vi "Set A4 Size.vi"(8 "error in (no error)":errorcluster, 10 "File refnum":refnum<k7>) -> (0 "error out":errorcluster, 2 "File refnum out":refnum<k7>)   [LabVIEW 2020, in "lvpptx.lvlib"]
uses:
  lvpptx.lvlib
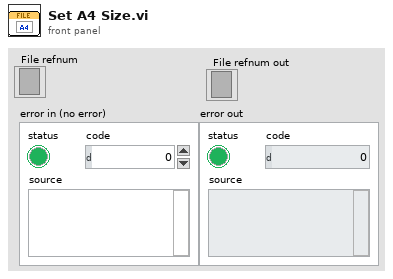
[diagram p1: front panel]
types:
  T1 = cluster{"SlideWidth (inches)":sgl, "SlideHeight (inches)":sgl}
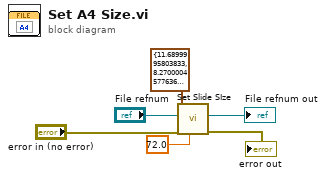
[diagram p0: block diagram]
diagram:
  n1 = call "Set Slide SIze.vi"("DPI"=72.0, "error in (no error)"="error in (no error)", "Slide size"=T1 {"SlideWidth (inches)"=11.69, "SlideHeight (inches)"=8.27}, "File refnum"="File refnum") -> ("error out"=→"error out":errorcluster, "File refnum out"=→"File refnum out":refnum<k7>)  [unwired: 6 in]
